vi "Get speed.vi"(11 "intake in":refnum<class "intake.lvclass">) -> (2 "speed":dbl, 3 "intake out":refnum<class "intake.lvclass">)   [LabVIEW 2015]
uses:
  intake.lvclass
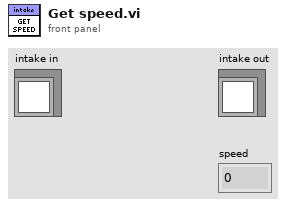
[diagram p1: front panel]
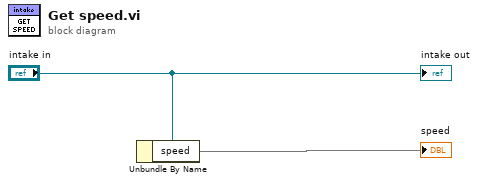
[diagram p0: block diagram]
diagram:
  n1 = Unbundle By Name("intake in") -> ("speed"=→"speed")
  "intake out" <- "intake in"
